vi "CreateProduct.vi"(8 "Error In":errorcluster, 11 "reference in":refnum<class "CarFactory.lvclass">) -> (0 "Error Out":errorcluster, 2 "ICarProduct":refnum<class "ICarProduct.lvclass">, 3 "reference out":refnum<class "CarFactory.lvclass">)   [LabVIEW 2024, in "CarFactory.lvclass"]
uses:
  CarFactory.lvclass
  CarFactory.lvclass/CarFactory.ctl
  ICarProduct/ICarProduct.lvclass
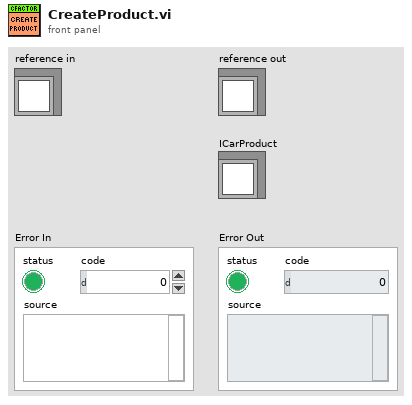
[diagram p1: front panel]
types:
  T1 = typedef "CarFactory.lvclass/ObjectAttributes.ctl" = cluster{"None":bool}
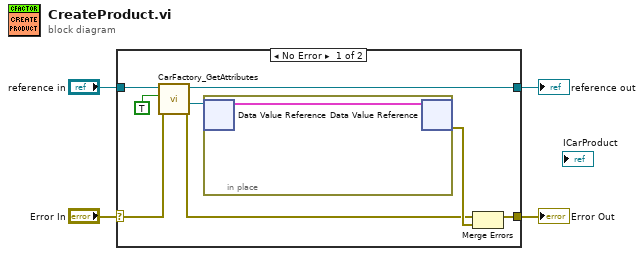
[diagram p0: block diagram]
diagram:
  n1 = case shown="No Error" "Error In" {
    selector: "Error In" -> [w11 w15]
    tunnel: [w8 w15] -> w3
    tunnel: [w9 w14] -> w1
    tunnel: "reference in" -> [w12 w14]
    frame No Error {
      n2 = call "CarFactory_GetAttributes.vi"("Error In"=w11, "OnlyGetDvrReference(False)"=TRUE, "reference in"=w12) -> ("Error Out"=w6:errorcluster, "DataRef"=w7:refnum<data-value>, "reference out"=w9:refnum<class "CarFactory.lvclass">)  [unwired: 5 in, 1 out]
      n3 = in-place {
        n4 = in-place-dvr #1(w7) -> (w13:T1)  [unwired: 1 out]
        n5 = in-place-dvr #1(w13) -> (w10:errorcluster)  [unwired: 1 out]
      }
      n6 = Merge Errors(w6, w10) -> (w8:errorcluster)
    }
    frame Error {
    }
  }
  "Error Out" <- w3
  "reference out" <- w1
